vi "Choreo_EventMarker_New.vi"(9 "Event":string, 11 "TimeStamp":dbl) -> (3 "EventMarker":T1)   [LabVIEW 2019, in "ChoreoLib.lvlib"]
doc: "Constructs an EventMarker with the specified parameters.\n\nInputs: \n -- timestamp - double - The timestamp of the event. (seconds)\n -- event - string - The event data string\n\nOutputs: \n -- EventMarker - cluster - the constructed event marker"
uses:
  ChoreoLib.lvlib
  TypeDef/ChoreoEventMarker.ctl
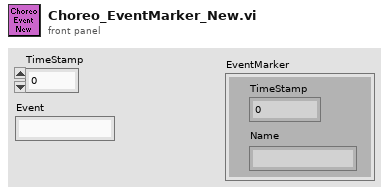
[diagram p1: front panel]
types:
  T1 = typedef "ChoreoLib.lvlib/ChoreoEventMarker.ctl" = cluster{"TimeStamp":dbl, "Name":string}
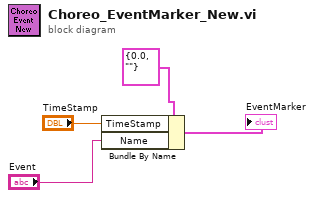
[diagram p0: block diagram]
diagram:
  n1 = Bundle By Name(cluster=T1 {"TimeStamp"=0.0, "Name"=""}, "TimeStamp"="TimeStamp", "Name"="Event") -> (→"EventMarker":T1)
